vi "Test Open Read Close WAV.vi"(8 "error in (no error)":errorcluster) -> (0 "error out":errorcluster, 3 "Pass?":bool)   [LabVIEW 2020]
uses:
  cad4d4b9-927c-4c9b-b99c-af13a2bbfaa3.vi
  G-Audio/Private/Get Basic Audio File Info.vi
  G-Audio/Private/Result To Error.vi
  cad4d4b9-927c-4c9b-b99c-af13a2bbfaa3.vi/779dfdfd-1b42-4cf4-8001-66d3dd167625.vi
  cad4d4b9-927c-4c9b-b99c-af13a2bbfaa3.vi/55d550d4-9624-414e-aebd-6e02b5081896.vi
  cad4d4b9-927c-4c9b-b99c-af13a2bbfaa3.vi/779dfdfd-1b42-4cf4-8001-66d3dd167625.vi/a9d2058a-38f9-4c88-a1a9-9bf864ebbde5.vi
  cad4d4b9-927c-4c9b-b99c-af13a2bbfaa3.vi/55d550d4-9624-414e-aebd-6e02b5081896.vi/4b7b629c-2e91-4160-9820-a26af8f6e677.vi
  cad4d4b9-927c-4c9b-b99c-af13a2bbfaa3.vi/55d550d4-9624-414e-aebd-6e02b5081896.vi/e7c4a249-ce38-42b4-8985-5fdb76b4ebfc.vi
  <vilib>/sound2/lvsound2.llb/Sound File Read Open.vi
  <vilib>/sound2/lvsound2.llb/Sound File Info (refnum).vi
  <vilib>/sound2/lvsound2.llb/Sound File Read (I16).vi
  <vilib>/Utility/Data Type/Get Numeric Information.vi
  <vilib>/Utility/error.llb/Error Cluster From Error Code.vi
  G-Audio/G-Audio.lvlib
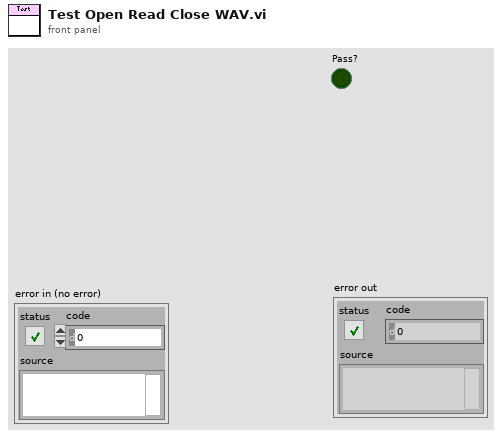
[diagram p1: front panel]
types:
  T1 = typedef "G-Audio.lvlib/Audio File Info.ctl" = cluster{"Sample Rate (Hz)":u32, "Channels":u32, "Bit Depth":u32}
  T2 = typedef "Sound File Refnum.ctl" = refnum<file>
  T3 = typedef "Sound Data Format.ctl" = cluster{"sample rate (S/s)":dbl, "number of channels":i32, "bits per sample":i32}
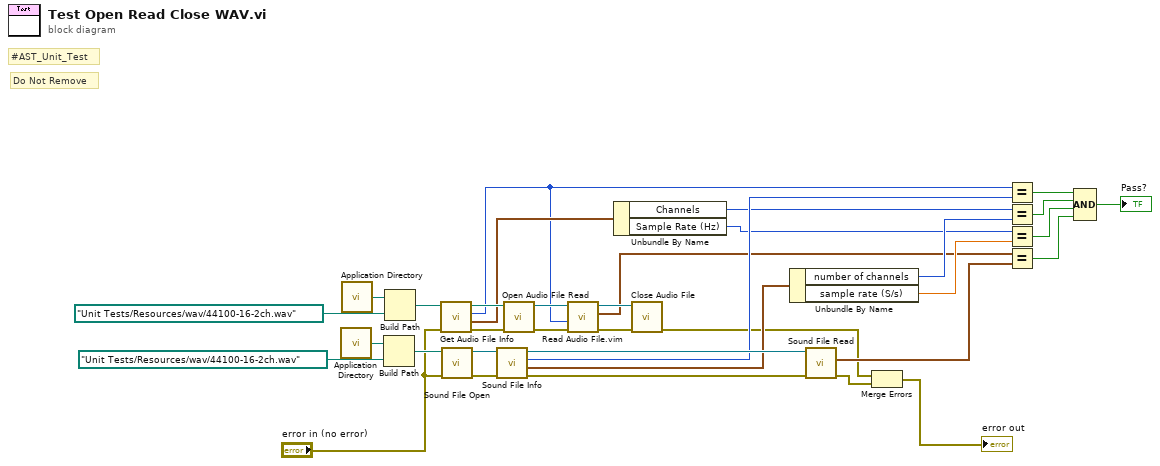
[diagram p0: block diagram]
diagram:
  # "Do Not Remove"
  # "#AST_Unit_Test"
  n1 = call <vilib>:"Application Directory.vi"() -> ("Application Directory"=w35:path)
  n2 = call <vilib>:"Application Directory.vi"() -> ("Application Directory"=w3:path)
  n3 = Build Path(base path=w35, name or relative path=path "Unit Tests/Resources/wav/44100-16-2ch.wav" ("Path")) -> (appended path=w34:path)
  n4 = Build Path(base path=w3, name or relative path=path "Unit Tests/Resources/wav/44100-16-2ch.wav" ("Path")) -> (appended path=w1:path)
  n5 = call "Get Audio File Info.vi"("error in (no error)"="error in (no error)", "Path In"=w1) -> ("error out"=w10:errorcluster, "Audio File Info"=w14:T1, "Sample Length"=w4:u64, "Path Out"=w16:path)  [unwired: 6 in]
  n6 = call-poly <vilib>:"Sound File Open.vi"("error in (no error)"="error in (no error)", "path"=w34) -> ("error out"=w23:errorcluster, "sound file refnum"=w32:T2)  [unwired: 8 in]
  n7 = call-poly <vilib>:"Sound File Info.vi"("error in (no error)"=w23, "sound file refnum"=w32) -> ("error out"=w22:errorcluster, "sound format"=w27:T3, "total number of samples/ch"=w28:u32, "sound file refnum out"=w31:T2)  [unwired: 6 in]
  n8 = call "Open Audio File Read.vi"("error in (no error)"=w10, "Path"=w16) -> ("error out"=w9:errorcluster, "Audio File Refnum"=w15:refnum<file>)  [unwired: 8 in]
  n9 = call "Read Audio File.vim"("error in (no error)"=w9, "Samples To Read"=w4, "Audio File Refnum In"=w15) -> ("error out"=w7:errorcluster, "Audio Data"=w5:waveform(i16)[], "Audio File Refnum Out"=w8:refnum<file>)  [unwired: 5 in, 1 out]
  n10 = Unbundle By Name(w14) -> ("Channels"=w13:u32, "Sample Rate (Hz)"=w12:u32)
  n11 = call "Close Audio File.vi"("error in (no error)"=w7, "Audio File Refnum In"=w8) -> ("error out"=w6:errorcluster)  [unwired: 9 in]
  n12 = Unbundle By Name(w27) -> ("number of channels"=w26:i32, "sample rate (S/s)"=w19:dbl)
  n13 = call-poly <vilib>:"Sound File Read.vi"("error in (no error)"=w22, "sound file refnum"=w31) -> ("error out"=w21:errorcluster, "data"=w18:waveform(i16)[])  [unwired: 5 in, 3 out]
  n14 = Merge Errors(w6, w21) -> (→"error out":errorcluster)
  n15 = Equal?(x=w4, y=w28) -> (x = y?=w30:bool)
  n16 = Equal?(x=w13, y=w26) -> (x = y?=w25:bool)
  n17 = Equal?(x=w12, y=w19) -> (x = y?=w24:bool)
  n18 = Equal?(x=w5, y=w18) -> (x = y?=w17:bool)
  n19 = Compound Arithmetic op=AND(w30, w25, w24, w17) -> (→"Pass?":bool)
